vi "Alarm Variable.vi"() -> ()   [LabVIEW 2010]
panel:
  out "Alarm Array":dbl[](array[numeric])
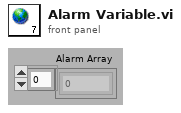
[diagram p1: front panel]
diagram:
